vi "_Remote Send Turbo Command 2.vi"(4 "error in (no error)":errorcluster, 7 "Telegram":string) -> (0 "error out":errorcluster, 3 "Raw Reply":string)   [LabVIEW 2012]
uses:
  Type/_RT Command.ctl
  Type/_RT Serial Command.ctl
panel:
  out "Hex Reply":string
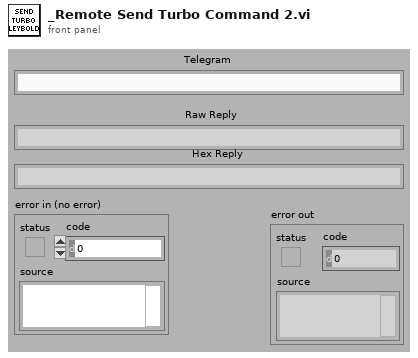
[diagram p1: front panel]
types:
  T1 = typedef "_RT Serial Command.ctl" = cluster{"Port Type":u16, "baud rate (9600)":u32, "data bits (8)":u16, "stop bits (1)":u16, "parity (0:none)":u16, "DoRead":bool, "Command":string}
  T2 = typedef "_RT Command.ctl" = enum16{"Start", "Stop", "Runtime Update", "Get Data", "Get Info", "Get Status", "Get Param", "Get Config", "Get Table", "Read ADC", "Set Oscillator", "Update Config", "Update Table", "Set All Pol", "Set Pol and DC", "Set Max Mass", "Toggle RP", "Toggle EL", "Set PIC", "Initialize Turbo", "Send Turbo Comm", "Close Turbo", "P1", "P2", "P3", "Send Serial", "Set LC Out", "Get LC In", "Read VAC", "Test Table", "Toggle Power", "Get Startup", "Set Startup", "Get ADC Table", "Set ADC Table", "Get Brief Status", "Get Detail Status", "Auxiliary Update", "Set CC Logics", "Set CC Input Logics", "Ignore Error"}
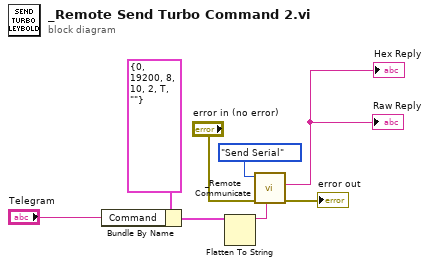
[diagram p0: block diagram]
diagram:
  n1 = Bundle By Name(cluster=T1 {"Port Type"=0, "baud rate (9600)"=19200, "data bits (8)"=8, "stop bits (1)"=10, "parity (0:none)"=2, "DoRead"=TRUE, "Command"=""} ("Serial Command"), "Command"="Telegram") -> (w5:T1)
  n2 = Flatten To String(anything=w5) -> (data string=w8:string)  [unwired: 1 in, 4 out]
  n3 = call "_Remote Communicate.vi"("String"=w8, "error in (no error)"="error in (no error)", "Command"=_RT_Command."Send Serial") -> ("error out"=→"error out":errorcluster, "Info"=→"Raw Reply" →"Hex Reply":string)  [unwired: 3 in, 2 out]
